vi "zad5_testowe.vi"() -> ()   [LabVIEW 2015]
panel:
  in  "Rozmiar tablicy N":dbl
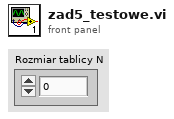
[diagram p1: front panel]
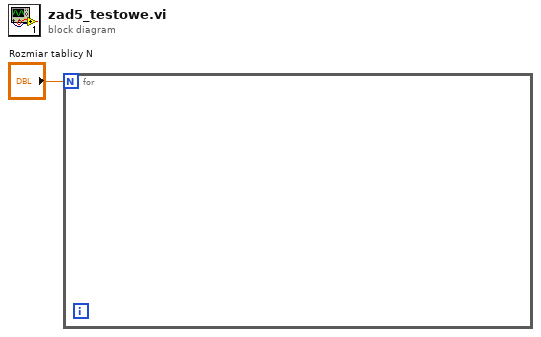
[diagram p0: block diagram]
diagram:
  n1 = for {
    N: "Rozmiar tablicy N" -> [_]
  }
